vi "Dialogue Box - Oscill Choice.vi"() -> ()   [LabVIEW 2020]
panel:
  out "Oscilloscope":u16(ring) items=["Lecroy 62xi", "Lecroy 64xi", "Lecroy 9300 series", ""]
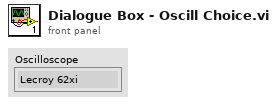
[diagram p1: front panel]
types:
  T1 = enum16{"Left Button", "Center Button", "Right Button", "Window Close"}
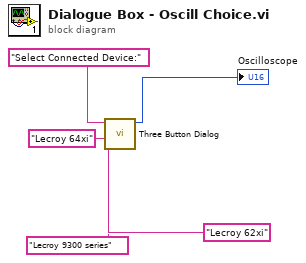
[diagram p0: block diagram]
diagram:
  n1 = call <vilib>:"Three Button Dialog.vi"("Right Button Text (\"Cancel\")"="Lecroy 9300 series" ("Right Button Text (\"Cancel\")"), "Center Button Text (\"No\")"="Lecroy 64xi" ("Center Button Text (\"No\")"), "Left Button Text (\"Yes\")"="Lecroy 62xi" ("Left Button Text (\"Yes\")"), "message"="Select Connected Device:") -> ("Which Button?"=→"Oscilloscope":T1)  [unwired: 7 in]
